vi "GenerationOnorOFF.vi"(8 "error in (no error)":errorcluster, 11 "ON/OFF":T1 items=["OFF", "ON"]) -> (0 "error out":errorcluster, 3 "ON/OFFCMD":string="SOUR:RFSG:GPRF:STAT ON")   [LabVIEW 2015]
uses:
  ONOFF.ctl
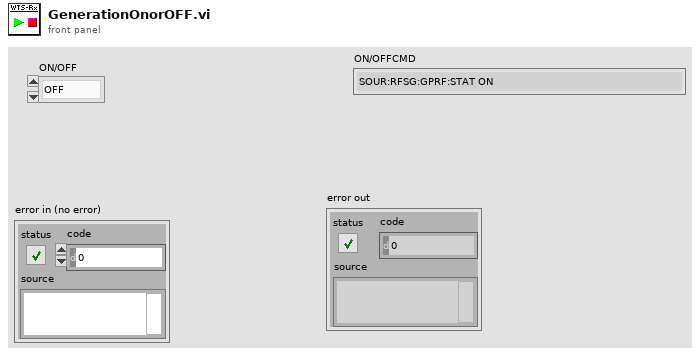
[diagram p1: front panel]
types:
  T1 = typedef "ONOFF.ctl" = u16
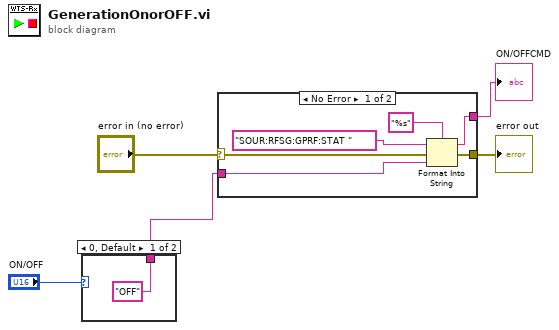
[diagram p0: block diagram]
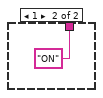
[diagram p2: hidden frame]
diagram:
  n1 = case shown="0, Default" "ON/OFF" {
    tunnel: ["OFF" ("ON/OFF") "ON" ("ON/OFF")] -> w1
    frame 0, Default {
    }
    frame 1 {
    }
  }
  n2 = case shown="No Error" "error in (no error)" {
    selector: "error in (no error)" -> [w9 w14]
    tunnel: w1 -> [w13 _]
    tunnel: [w10 _] -> w5
    tunnel: [w8 w14] -> w3
    frame No Error {
      n3 = Format Into String(format string="%s", initial string="SOUR:RFSG:GPRF:STAT ", error in=w9, w13) -> (resulting string=w10:string, error out=w8:errorcluster)
    }
    frame Error {
    }
  }
  "ON/OFFCMD" <- w5
  "error out" <- w3
